vi "Algo_Sequence.vi"(7 "Array of Input Values":dbl[](array[numeric]), 8 "error in (no error)":errorcluster, 9 "Array of Math Expression":string[](array[string])=["c = 2*a + 3*b", "d = 3*sin(0) + 4*cos(0)", "e = 4*a + 5*b", "f = 4*a + 5*b", "g = 4*a + 5*b", "h = 4*a + 5*b", "i = 4*a + 5*b", "j = 4*a + 5*b", "j = 4*a + 5*b", "k = 4*a + 5*b"], 10 "Array of Result Variables Out":string[](array[string]), 11 "Array of Result Variables In":string[](array[string])) -> (0 "error out":errorcluster, 3 "Array of Final Results":dbl[](array[numeric]))   [LabVIEW 2019, in "Algorithm.lvclass"]
uses:
  FrameworkOverrides/Algorithm.lvclass
  <vilib>/gmath/NI_Gmath.lvlib
panel:
  out "Output Values":dbl[][](array[numeric])
  out "Array 2":i32[](array[numeric])
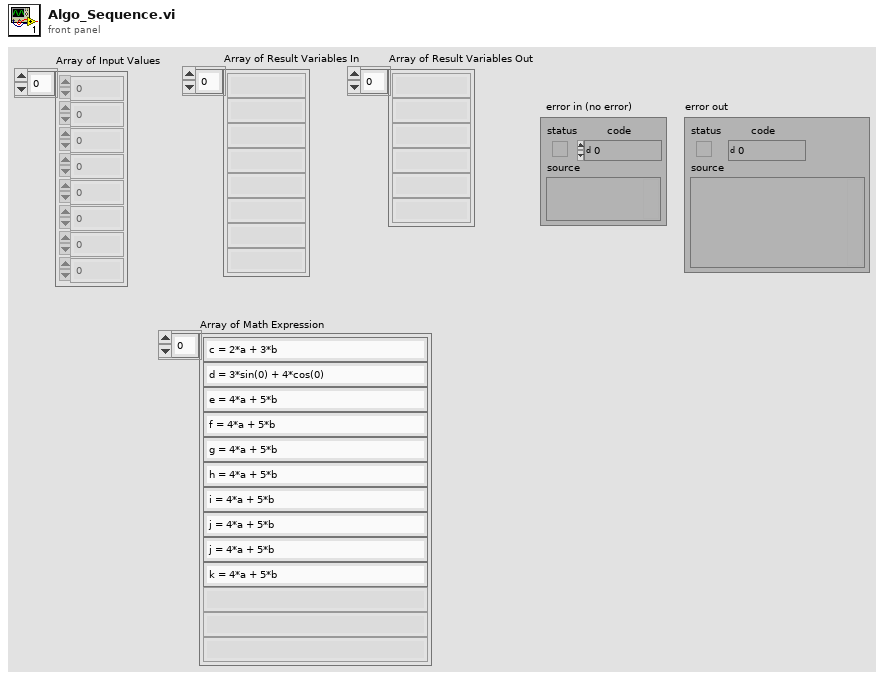
[diagram p1: front panel]
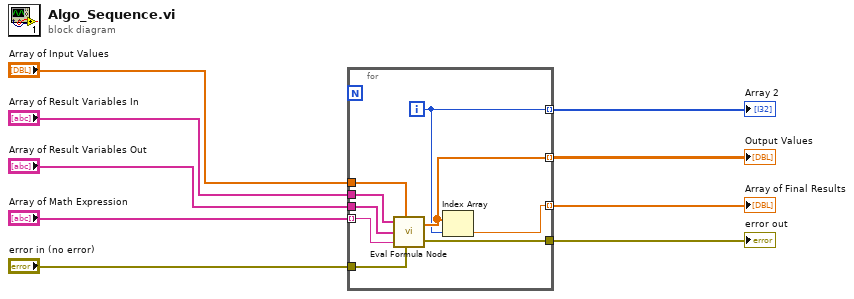
[diagram p0: block diagram]
diagram:
  n1 = for {
    tunnel: "Array of Result Variables In" -> [w18]
    tunnel: "Array of Result Variables Out" -> [w17]
    tunnel: "Array of Input Values" -> [w16]
    tunnel: [w12] -> w8 mode=indexing
    tunnel: "Array of Math Expression" -> [w13] mode=indexing
    tunnel: [w11] -> w9 mode=indexing
    tunnel: "error in (no error)" -> [w15]
    tunnel: [w14] -> w5
    tunnel: [w10] -> w7 mode=indexing
    i -> [w11]
    n2 = call <vilib>:"Eval Formula Node.vi"("Variables Input"=w18, "Input Values"=w16, "Variables Output"=w17, "formula"=w13, "error in (no error)"=w15) -> ("Output Values"=w12:dbl[], "error out"=w14:errorcluster)
    n3 = Index Array(array=w12, index=w11) -> (element=w10:dbl)
  }
  "Array 2" <- w9
  "Output Values" <- w8
  "Array of Final Results" <- w7
  "error out" <- w5
